vi "StopLDOTest.vi"(8 "error in (no error)":errorcluster, 11 "Queue in":refnum<queue>) -> (0 "error out":errorcluster)   [LabVIEW 2020]
uses:
  support/Message Queue/Message Cluster.ctl
  support/Message Queue/Enqueue Message (Single).vi
  support/Message Queue/Message Queue.lvlib
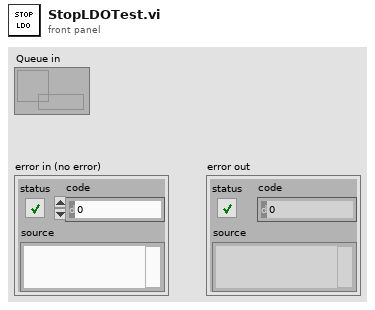
[diagram p1: front panel]
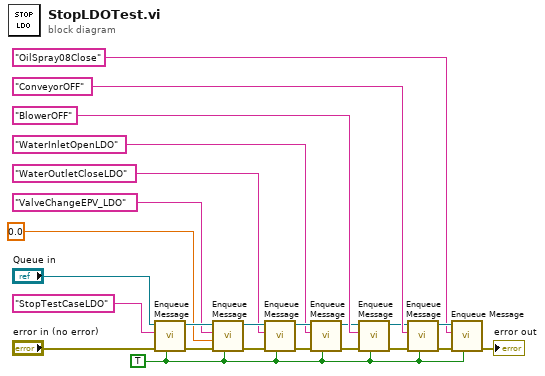
[diagram p0: block diagram]
diagram:
  w1 = TRUE ("Priority Message? (F)")
  n1 = call-poly "Enqueue Message.vi"("Priority Message? (F)"=w1, "error in (no error)"="error in (no error)", "Message"="StopTestCaseLDO", "Message Queue"="Queue in") -> ("error out"=w9:errorcluster, "dup Message Queue"=w8:refnum<queue>)  [unwired: 6 in]
  n2 = call-poly "Enqueue Message.vi"("Priority Message? (F)"=w1, "error in (no error)"=w9, "Message Data"=0.0 ("Proportioning Valve 2"), "Message"="ValveChangeEPV_LDO", "Message Queue"=w8) -> ("error out"=w11:errorcluster, "dup Message Queue"=w12:refnum<queue>)  [unwired: 5 in]
  n3 = call-poly "Enqueue Message.vi"("Priority Message? (F)"=w1, "error in (no error)"=w11, "Message"="WaterOutletCloseLDO", "Message Queue"=w12) -> ("error out"=w14:errorcluster, "dup Message Queue"=w15:refnum<queue>)  [unwired: 6 in]
  n4 = call-poly "Enqueue Message.vi"("Priority Message? (F)"=w1, "error in (no error)"=w14, "Message"="WaterInletOpenLDO", "Message Queue"=w15) -> ("error out"=w20:errorcluster, "dup Message Queue"=w2:refnum<queue>)  [unwired: 6 in]
  n5 = call-poly "Enqueue Message.vi"("Priority Message? (F)"=w1, "error in (no error)"=w20, "Message"="BlowerOFF", "Message Queue"=w2) -> ("error out"=w17:errorcluster, "dup Message Queue"=w16:refnum<queue>)  [unwired: 6 in]
  n6 = call-poly "Enqueue Message.vi"("Priority Message? (F)"=w1, "error in (no error)"=w17, "Message"="ConveyorOFF", "Message Queue"=w16) -> ("error out"=w23:errorcluster, "dup Message Queue"=w22:refnum<queue>)  [unwired: 6 in]
  n7 = call-poly "Enqueue Message.vi"("Priority Message? (F)"=w1, "error in (no error)"=w23, "Message"="OilSpray08Close", "Message Queue"=w22) -> ("error out"=→"error out":errorcluster)  [unwired: 6 in, 1 out]
